vi "Evaluate Test.vi"(7 "Test Executive Ref out":refnum<data-value>, 11 "Executioner in":refnum<class "Executioner.lvclass">) -> (3 "Value":i32)   [LabVIEW 2020, in "Test Executive.lvlib" / "Mock Executioner.lvclass"]
uses:
  <vilib>/gpm_packages/@cs/test-executive/Source/Sandbox/While Loop Stop Example/Mock Executioner/Mock Executioner.lvclass
  <vilib>/gpm_packages/@cs/test-executive/Source/Test Executive/Executioner/Executioner.lvclass
  <vilib>/gpm_packages/@cs/test-executive/Source/Test Executive/ITestExecutive/ITest Executive.lvclass
  <vilib>/gpm_packages/@cs/lookup-table/Source/LookupTable/LookupTable.lvclass/LookupTable.ctl
  ac680d32-2ae2-49fb-88bb-a405b46d6c82.vi
  3a6a9cdd-5029-414c-aee1-24faa3875e61.vi
  992808d7-9fcb-4807-9aa6-d42f2418f55a.vi
  <vilib>/gpm_packages/@cs/lookup-table/Source/LookupTable/Read Table Reference.vi
  ac680d32-2ae2-49fb-88bb-a405b46d6c82.vi/3de0621f-49a0-4449-9f54-796c7cfeda1f.vi
  <vilib>/Utility/error.llb/Error Cluster From Error Code.vi
  <vilib>/gpm_packages/@cs/lookup-table/Source/LookupTable/LookupTable.lvclass
  <vilib>/gpm_packages/@cs/test-executive/Source/Test Executive/TestExecutive Ref/TestExecutive Ref.lvclass
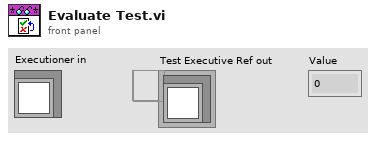
[diagram p1: front panel]
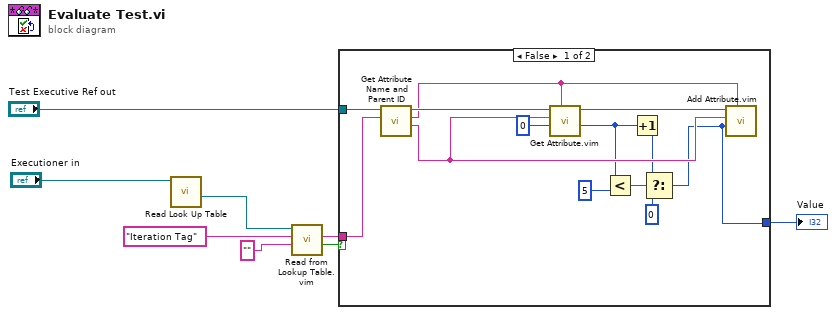
[diagram p0: block diagram]
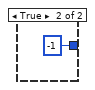
[diagram p2: hidden frame]
diagram:
  n1 = call <vilib>:"Read Look Up Table.vi"("Executioner in"="Executioner in") -> ("Attributes Ref"=w1:refnum<data-value>)  [unwired: 9 in, 1 out]
  n2 = call "Read from Lookup Table.vim"("Type"="", "Item Name"="Iteration Tag", "LookupTable Reference"=w1) -> ("Not Found?"=w3:bool, "Value"=w6:string)  [unwired: 5 in, 2 out]
  n3 = case shown="False" w3 {
    tunnel: "Test Executive Ref out" -> [w21 _]
    tunnel: w6 -> [w15 _]
    tunnel: [w9 -1] -> w4
    frame False {
      n4 = call <vilib>:"Get Attribute Name and Parent ID.vi"("Tag"=w15, "Test Executive Ref"=w21) -> ("Attribute Name"=w16:string, "Parent ID"=w17:string, "Test Executive Ref out"=w20:refnum<data-value>)  [unwired: 6 in, 1 out]
      n5 = call "Get Attribute.vim"("ID"=w17, "Type"=0, "Attribute Name"=w16, "Test Executive Ref"=w20) -> ("Attribute"=w14:i32, "Test Executive Ref out"=w18:refnum<data-value>)  [unwired: 3 in, 3 out]
      n6 = Less?(x=w14, y=5) -> (x < y?=w12:bool)
      n7 = Increment(x=w14) -> (x+1=w10:i32)
      n8 = Select(t=w10, s=w12, f=0) -> (s? t:f=w9:i32)
      n9 = call "Add Attribute.vim"("ID"=w17, "Attribute"=w9, "Attribute Name"=w16, "Test Executive Ref"=w18) -> ()  [unwired: 4 in, 4 out]
    }
    frame True {
    }
  }
  "Value" <- w4
